vi "Get Baratron Voltage.vi"(8 "error in (no error)":errorcluster, 10 "Baratron Voltage":waveform(dbl)[](array[waveform]), 11 "Baratron in":refnum<class "Baratron.lvclass">) -> (0 "error out":errorcluster, 3 "Baratron out":refnum<class "Baratron.lvclass">)   [LabVIEW 2021, in "Baratron.lvlib" / "Baratron.lvclass"]
uses:
  Baratron.lvclass
  C:/Program Files/National Instruments/LabVIEW 2021/vi.lib/ActorFramework/Actor/Actor.lvclass
  Baratron.lvclass/Baratron.ctl
  <vilib>/ActorFramework/Actor/Actor.lvclass/Actor.ctl
  Baratron Pressure/Baratron Pressure Messages/Baratron Pressure Msg/Baratron Pressure Msg.lvclass/Baratron Pressure Msg.ctl
  <vilib>/ActorFramework/Message Enqueuer/Message Enqueuer.lvclass/Message Enqueuer.ctl
  <vilib>/ActorFramework/Message Enqueuer/Enqueue.vi
  Baratron Pressure/Baratron Pressure Messages/Baratron Pressure Msg/Baratron Pressure Msg.lvclass
  C:/Program Files/National Instruments/LabVIEW 2021/vi.lib/ActorFramework/Message/Message.lvclass
  <vilib>/ActorFramework/Message Priority Queue/Priority Enqueue.vi
  DAQ-arch/Analog Input Publisher/Analog Input Publisher.lvclass
  <vilib>/ActorFramework/Actor/Actor.lvclass
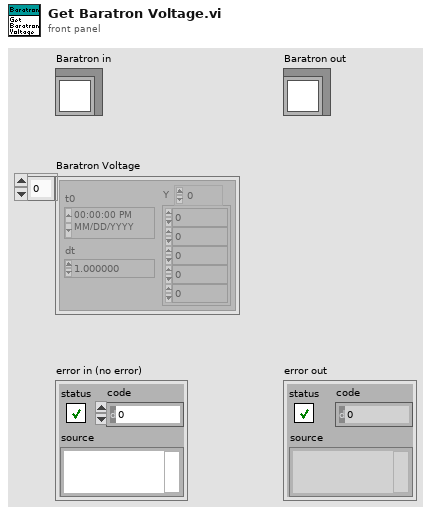
[diagram p1: front panel]
types:
  T1 = typedef "Baratron.lvlib/Baratron.lvclass/Status Range.ctl" = enum16{"Above Range", "Below Range", "Within Range"}
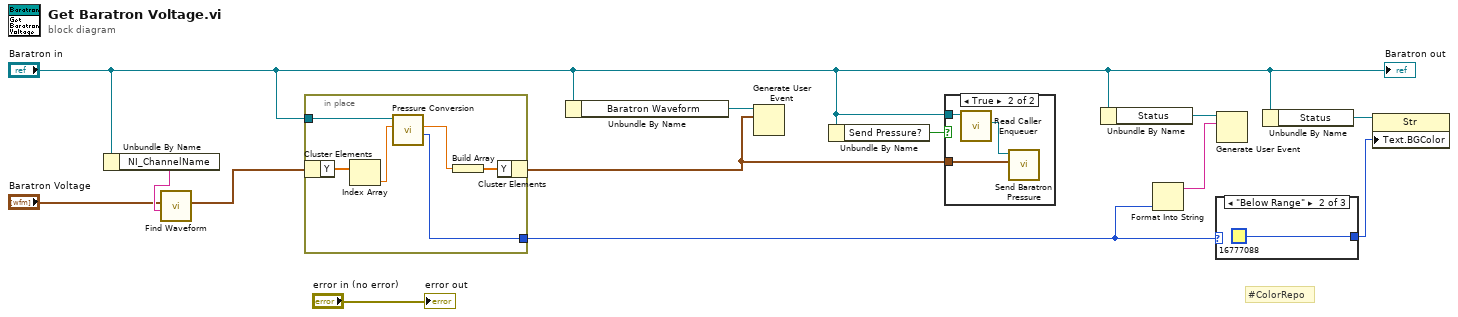
[diagram p0: block diagram]
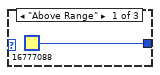
[diagram p3: hidden frame]
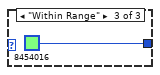
[diagram p4: hidden frame]
diagram:
  # "#ColorRepo"
  n1 = Unbundle By Name("Baratron in") -> ("NI_ChannelName"=w6:string)
  n2 = call "Find Waveform.vi"("NI_ChannelName"=w6, "Waveform"="Baratron Voltage") -> ("Last Waveform"=w5:waveform(dbl))  [unwired: 8 in, 1 out]
  n3 = in-place {
    in-place-border: [w16] -> w8
    in-place-border: "Baratron in" -> [w15]
    n4 = in-place-cluster #1(w5) -> ("Y"=w17:dbl[])
    n5 = Index Array(array=w17) -> (element=w18:dbl)  [unwired: 1 in]
    n6 = call "Pressure Conversion.vi"("Voltage"=w18, "Baratron in"=w15) -> ("Status Range"=w16:T1, "Pressure"=w14:dbl)  [unwired: 8 in]
    n7 = Build Array(w14) -> (w19:dbl[])
    n8 = in-place-cluster #1("Y"=w19) -> (w3:waveform(dbl))
  }
  n9 = Unbundle By Name("Baratron in") -> ("Baratron Waveform"=w12:refnum<user-event>)
  n10 = Generate User Event(user event=w12, event data cluster=w3) -> ()  [unwired: 2 in, 2 out]
  n11 = Unbundle By Name("Baratron in") -> ("Send Pressure?"=w4:bool)
  n12 = case shown="True" w4 {
    tunnel: "Baratron in" -> [_ w21]
    tunnel: w3 -> [_ w20]
    frame False {
    }
    frame True {
      n13 = call <vilib>:"Read Caller Enqueuer.vi"("Actor"=w21) -> ("Caller Enqueuer"=w22:refnum<class "Message Enqueuer.lvclass">)  [unwired: 10 in]
      n14 = call "Send Baratron Pressure.vi"("Baratron Pressure"=w20, "Message Enqueuer"=w22) -> ()  [unwired: 8 in, 2 out]
    }
  }
  n15 = Unbundle By Name("Baratron in") -> ("Status"=w10:refnum<user-event>)
  n16 = Format Into String(w8) -> (resulting string=w9:string)  [unwired: 3 in, 1 out]
  n17 = case shown="\"Below Range\"" w8 {
    tunnel: [u32 16777088 ("Text.Colors:BG Color") u32 16777088 ("Text.Colors:BG Color") u32 8454016 ("Text.Colors:BG Color")] -> w7
    frame "Above Range" {
    }
    frame "Below Range" {
    }
    frame "Within Range" {
    }
  }
  n18 = Generate User Event(user event=w10, event data cluster=w9) -> ()  [unwired: 2 in, 2 out]
  n19 = Unbundle By Name("Baratron in") -> ("Status"=w11:refnum<vi>)
  n20 = property class="Str"(reference=w11, "Text.BGColor"=w7) -> ()  [unwired: 1 in, 2 out]
  "error out" <- "error in (no error)"
  "Baratron out" <- "Baratron in"
